vi "solar_voy_def Resolve ASCII (Hex).vi"(10 "DEFAULT (ASCII '\\xFF')":string) -> (2 "Resolved DEFAULT (Hex 'xFF')":string)   [LabVIEW 2018]
doc: "This converts a hexidecimal string ('\\xFF\\x02\\x..') to value."
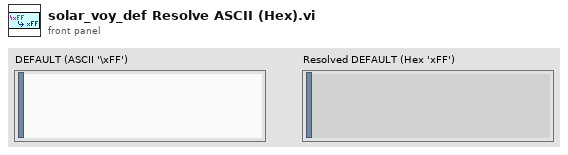
[diagram p1: front panel]
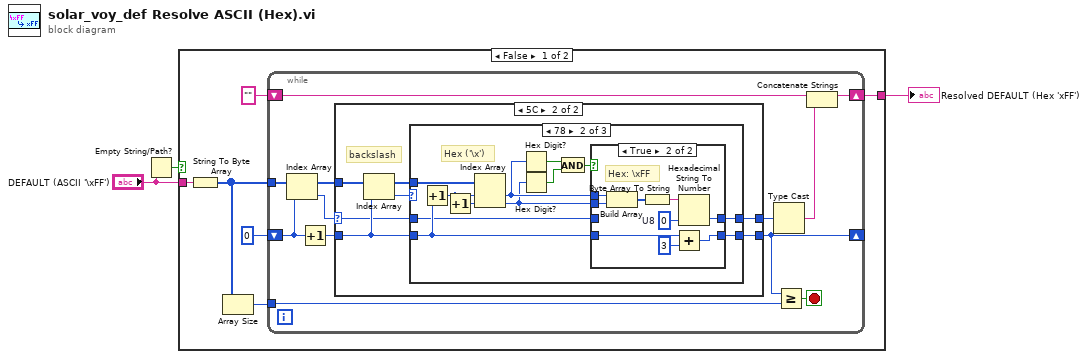
[diagram p0: block diagram]
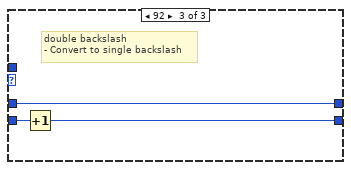
[diagram p5: hidden frame]
diagram:
  n1 = Empty String/Path?(string/path="DEFAULT (ASCII '\\xFF')") -> (empty?=w1:bool)
  n2 = case shown="False" w1 {
    tunnel: "DEFAULT (ASCII '\\xFF')" -> [w9 _]
    tunnel: [w5 _] -> w3
    frame False {
      n3 = String To Byte Array(string=w9) -> (unsigned byte array=w8:u8[])
      n4 = Array Size(array=w8) -> (size(s)=w4:i32)
      n5 = while {
        tunnel: w8 -> [w20]
        shift-right: [w13] -> _
        shift-left: 0 -> [w19]
        shift-right: [w15] -> w5
        shift-left: "" -> [w16]
        tunnel: w4 -> [w12]
        stop <- w11 stop-if-true
        n6 = Index Array(array=w20, index=w19) -> (element=w10:u8)
        n7 = Increment(x=w19) -> (x+1=w18:i32)
        n8 = case shown="5C" w10 {
          selector: w10 -> [w21 w24]
          tunnel: w20 -> [_ w27]
          tunnel: w18 -> [w22 w26]
          tunnel: [w22 w25] -> w13
          tunnel: [w21 w23] -> w17
          frame Default {
          }
          frame 92 {
            # "backslash"
            n9 = Index Array(array=w27, index=w26) -> (element=w28:u8)
            n10 = case shown="78" w28 {
              tunnel: w27 -> [_ w42 _]
              tunnel: w26 -> [w30 w34 w56]
              tunnel: [w30 w33 w54] -> w25
              tunnel: w24 -> [w29 w32 w55]
              tunnel: [w29 w31 w55] -> w23
              frame Default {
              }
              frame 120 {
                # "Hex ('\\x')"
                n11 = Increment(x=w34) -> (x+1=w41:i32)
                n12 = Increment(x=w41) -> (x+1=w40:i32)
                n13 = Index Array(array=w42, index #1=w41, index #2=w40) -> (element #1=w36:u8, element #2=w35:u8)
                n14 = Hex Digit?(1:w36) -> (0:w39:bool)
                n15 = Hex Digit?(1:w35) -> (0:w38:bool)
                n16 = And(x=w39, y=w38) -> (x .and. y?=w37:bool)
                n17 = case shown="True" w37 {
                  tunnel: w36 -> [_ w53]
                  tunnel: w35 -> [_ w52]
                  tunnel: w34 -> [w44 w48]
                  tunnel: [w44 w46] -> w33
                  tunnel: [w43 w45] -> w31
                  tunnel: w32 -> [w43 _]
                  frame False {
                  }
                  frame True {
                    w49 = u8 0  # U8
                    # "Hex: \\xFF"
                    n18 = Build Array(w53, w52) -> (w51:u8[])
                    n19 = Byte Array To String(unsigned byte array=w51) -> (string=w50:string)
                    n20 = Add(x=w48, y=3) -> (x+y=w46:i32)
                    n21 = Hexadecimal String To Number(string=w50, default (0uL)=w49) -> (number=w45:u8)  [unwired: 1 in, 1 out]
                  }
                }
              }
              frame 92 {
                # "double backslash\n- Convert to single backslash"
                n22 = Increment(x=w56) -> (x+1=w54:i32)
              }
            }
          }
        }
        n23 = Type Cast(x=w17) -> (*(type *) &x=w14:string)  [unwired: 1 in]
        n24 = Greater Or Equal?(x=w13, y=w12) -> (x >= y?=w11:bool)
        n25 = Concatenate Strings(w16, w14) -> (w15:string)
      }
    }
    frame True {
    }
  }
  "Resolved DEFAULT (Hex 'xFF')" <- w3
